vi "Make RR JSON.vi"(9 "Force":bool, 10 "roboRIO prev":T1={"type"="roboRIO", "device"="", "name"="", "data"={">fpga_button"=FALSE, ">vin_voltage"=0.0, ">vin_current"=0.0, ">6v_voltage"=0.0, ">6v_current"=0.0, ">6v_active"=FALSE, ">6v_faults"=0.0, ">5v_voltage"=0.0, ">5v_current"=0.0, ">5v_active"=FALSE, ">5v_faults"=0.0, ">3v3_voltage"=0.0, ">3v3_current"=0.0, ">3v3_active"=FALSE, ">3v3_faults"=0.0}}, 11 "roboRIO new":T1={"type"="roboRIO", "device"="", "name"="", "data"={">fpga_button"=FALSE, ">vin_voltage"=0.0, ">vin_current"=0.0, ">6v_voltage"=0.0, ">6v_current"=0.0, ">6v_active"=FALSE, ">6v_faults"=0.0, ">5v_voltage"=0.0, ">5v_current"=0.0, ">5v_active"=FALSE, ">5v_faults"=0.0, ">3v3_voltage"=0.0, ">3v3_current"=0.0, ">3v3_active"=FALSE, ">3v3_faults"=0.0}}) -> (3 "delta JSON":string)   [LabVIEW 2019]
uses:
  RoboRIO proto.ctl
  RoboRIO data proto.ctl
panel:
  out "Complete JSON":string
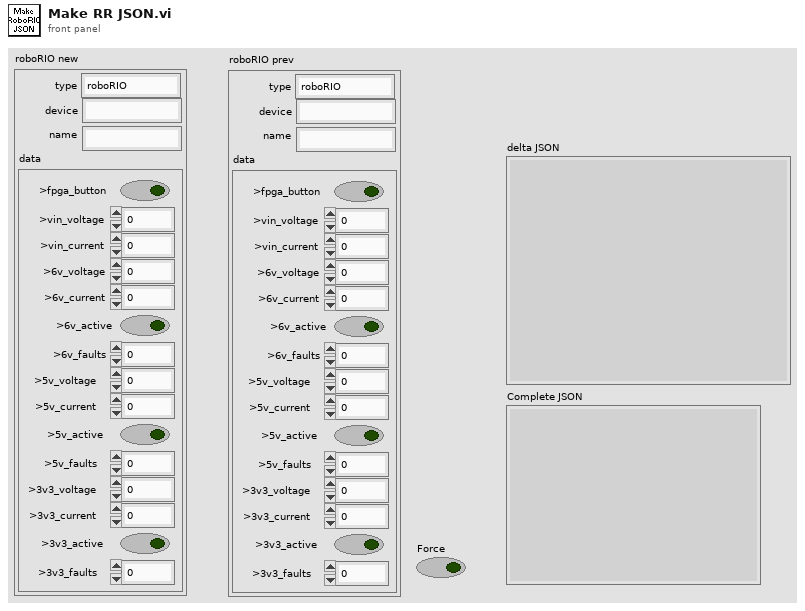
[diagram p1: front panel]
types:
  T1 = typedef "RoboRIO proto.ctl" = cluster{"type":string, "device":string, "name":string, "data":T2}
  T2 = typedef "RoboRIO data proto.ctl" = cluster{">fpga_button":bool, ">vin_voltage":dbl, ">vin_current":dbl, ">6v_voltage":dbl, ">6v_current":dbl, ">6v_active":bool, ">6v_faults":dbl, ">5v_voltage":dbl, ">5v_current":dbl, ">5v_active":bool, ">5v_faults":dbl, ">3v3_voltage":dbl, ">3v3_current":dbl, ">3v3_active":bool, ">3v3_faults":dbl}
  T3 = cluster{"type":bool, "device":bool, "name":bool, "data":cluster{">fpga_button":bool, ">vin_voltage":bool, ">vin_current":bool, ">6v_voltage":bool, ">6v_current":bool, ">6v_active":bool, ">6v_faults":bool, ">5v_voltage":bool, ">5v_current":bool, ">5v_active":bool, ">5v_faults":bool, ">3v3_voltage":bool, ">3v3_current":bool, ">3v3_active":bool, ">3v3_faults":bool}}
  T4 = cluster{">fpga_button":bool, ">vin_voltage":bool, ">vin_current":bool, ">6v_voltage":bool, ">6v_current":bool, ">6v_active":bool, ">6v_faults":bool, ">5v_voltage":bool, ">5v_current":bool, ">5v_active":bool, ">5v_faults":bool, ">3v3_voltage":bool, ">3v3_current":bool, ">3v3_active":bool, ">3v3_faults":bool}
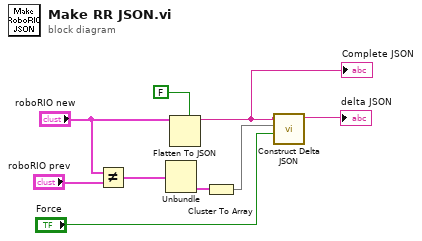
[diagram p0: block diagram]
diagram:
  n1 = Not Equal?(x="roboRIO new", y="roboRIO prev") -> (x != y?=w1:T3)
  n2 = Unbundle(w1) -> ("data"=w3:T4)  [unwired: 3 out]
  n3 = Flatten To JSON(enable LabVIEW extensions? (T)=FALSE, anything="roboRIO new") -> (JSON string=w6:string)  [unwired: 1 in, 1 out]
  "Complete JSON" <- w6
  n4 = Cluster To Array(cluster=w3) -> (array=w2:bool[])
  n5 = call "Construct Delta JSON.vi"("Force"="Force", "Checked Items"=w2, "JSON string"=w6) -> ("Delta JSON"=→"delta JSON":string)  [unwired: 8 in]
